vi "FloatingMean_Example.vi"() -> ()   [LabVIEW 2019]
doc: "This example shows how to compute and show a floating mean live image.\nHere the camera class is operated in fifo mode to always get next image in buffer.\nThe Average Count defines the number of images that will be averaged.\nAveraging is done by fetiching one image and using average image from previous iteration\n(avg_n = (1-1/avg_count)*avg_(n-1) + (1/avg_count)*image_n)\n\nIt is a good starting point for writing own applications.\nBut it will not be fail save, i.e. doesnt react on errors, just handles them forward to the end\n\nUsage:\nSelect your required fifo buffer size and image format and start the program.\nOnce started, the camera class will be initialized and image record will start automatically.\nInside the acquisition loop the program calculates the floating average image shows it.\nThe average count can be changed at any time.\nBy using the ROI parameters you can crop the image to select certain regions\n\nBy clicking Quit Application the record will stop and will force an exit of the camera class"
uses:
  camera/Camera.lvclass
  <vilib>/picture/picture.llb/Draw True-Color Pixmap.vi
  <vilib>/picture/picture.llb/Draw 8-Bit Pixmap.vi
panel:
  out "colormap(U8)":u32[](array[numeric])
  in  "Zoom [%]":i32(slide)=26 min=10 max=200 step=5 scale=10.0..200.0
  out "Image":picture
  out "Image(U16)":u16[][](graph)
  in  "averageCount":u8=10 caption="Average Count" min=2
  in  "data_format":T1(ring)=enum."Mono16"
  out "Recorded Images":u32
  in  "Quit":bool
  in  "cropY1":u64=2048 min=1 max=2048 step=1
  in  "cropX1":u64=2048 min=1 max=2048 step=1
  in  "cropY0":u64=1 min=1 max=2047 step=1
  in  "cropX0":u64=1 min=1 max=2047 step=1
  out "Image Height":u64
  out "Image Width":u64
  in  "dwImgCount":u32=10 caption="Fifo Buffer Size" max=4023
  out "Error":errorcluster {"code" format="%x"}
  # "This example shows how to compute and show a floating mean live image.\nHere the camera class is operated in fifo mode to always get next image in buffer.\nThe Average Count defines the number of images that will be averaged.\nAveraging is done by fetiching one image and using average image from previous iteration\n(avg_n = (1-1/avg_count)*avg_(n-1) + (1/avg_count)*image_n)\n\nIt is a good starting point for writing own applications.\nBut it will not be fail save, i.e. doesnt react on errors, just handles them forward to the end\n\nUsage:\nSelect your required fifo buffer size and image format and start the program.\nOnce started, the camera class will be initialized and image record will start automatically.\nInside the acquisition loop the program calculates the floating average image shows it.\nThe average count can be changed at any time.\nBy using the crop parameters you can crop the image to select certain regions\n\nBy clicking Quit Application the record will stop and will force an exit of the camera class"
  # "pco.labview"
  # "Camera Setup"
  # "Recording Control"
  # "Parameters for image readout"
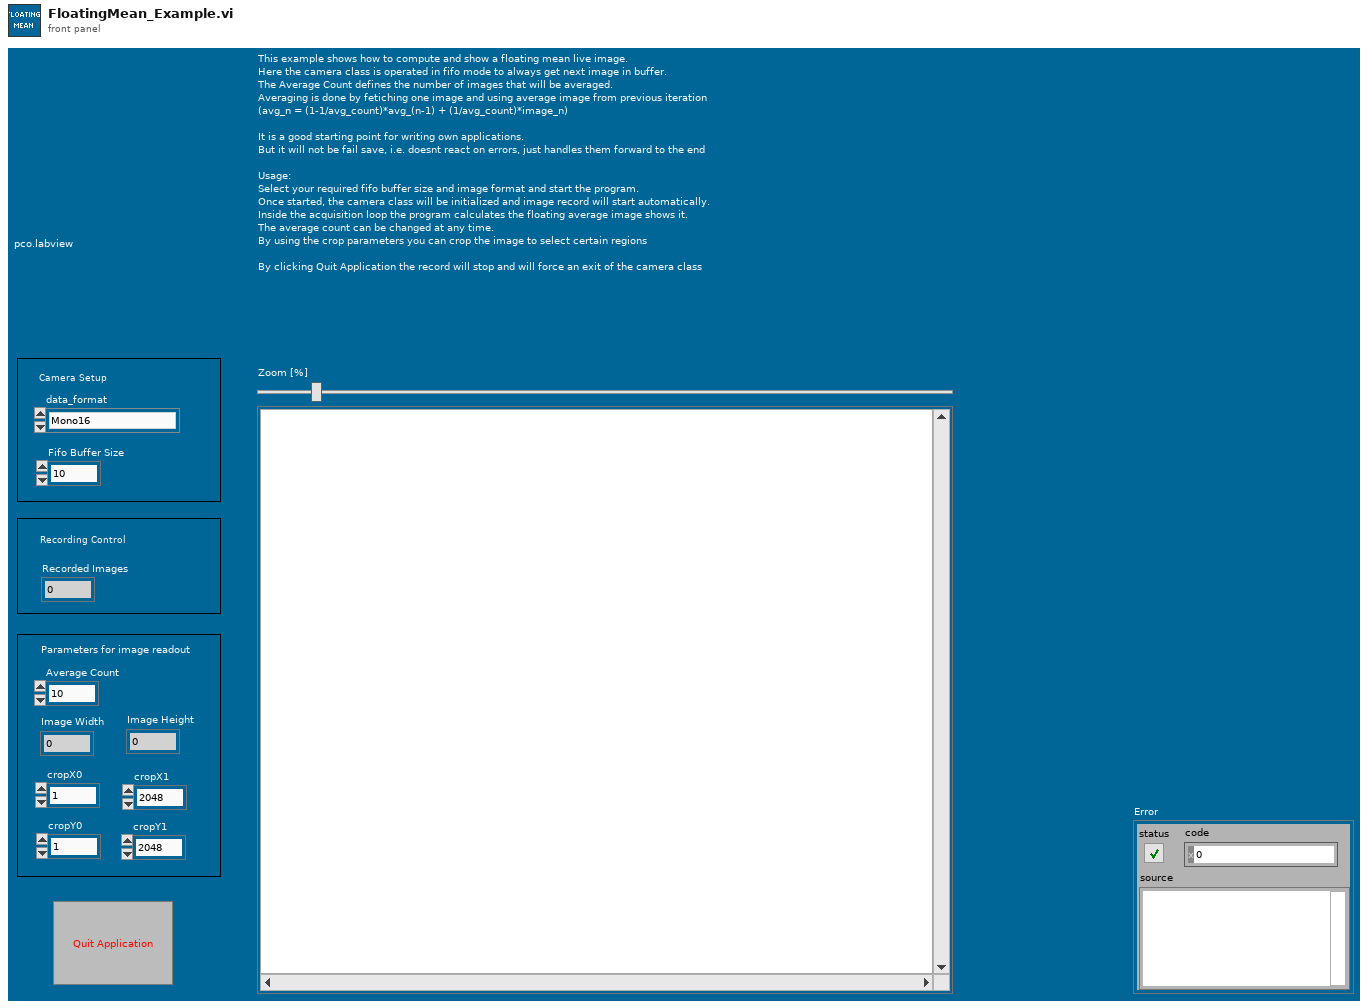
[diagram p1: front panel]
types:
  T1 = enum16{"Undefined", "Mono8", "Mono16", "BGRA8", "RGBA8", "BGRA16", "RGBA16", "CompressedMono8"}
  T2 = enum8{"Enabled", "Disabled", "Disabled and Grayed Out"}
  T3 = enum16{"sequence", "sequence non blocking", "ring buffer", "fifo", "tif", "multitif", "pcoraw", "b16", "dicom", "multidicom", "camram_ring", "camram_segment"}
  T4 = typedef "Camera.lvclass/binning.ctl" = cluster{"vert":u16, "horz":u16, "mode":u16}
  T5 = cluster{"exposure_time_s":dbl, "delay_time_s":dbl, "roi":cluster{"x0":u64, "y0":u64, "x1":u64, "y1":u64}, "timestamp_mode":u16, "pixelrate":u32, "conversion_factor":sgl, "trigger_mode":u16, "acquire_mode":u16, "acquire_sequence_number":u32, "metadata_mode":u16, "noisefilter_mode":u16, "pixel_format":u32, "binning":T4, "auto_exposure":cluster{"region":u16, "min_exposure_s":dbl, "max_exposure_s":dbl}}
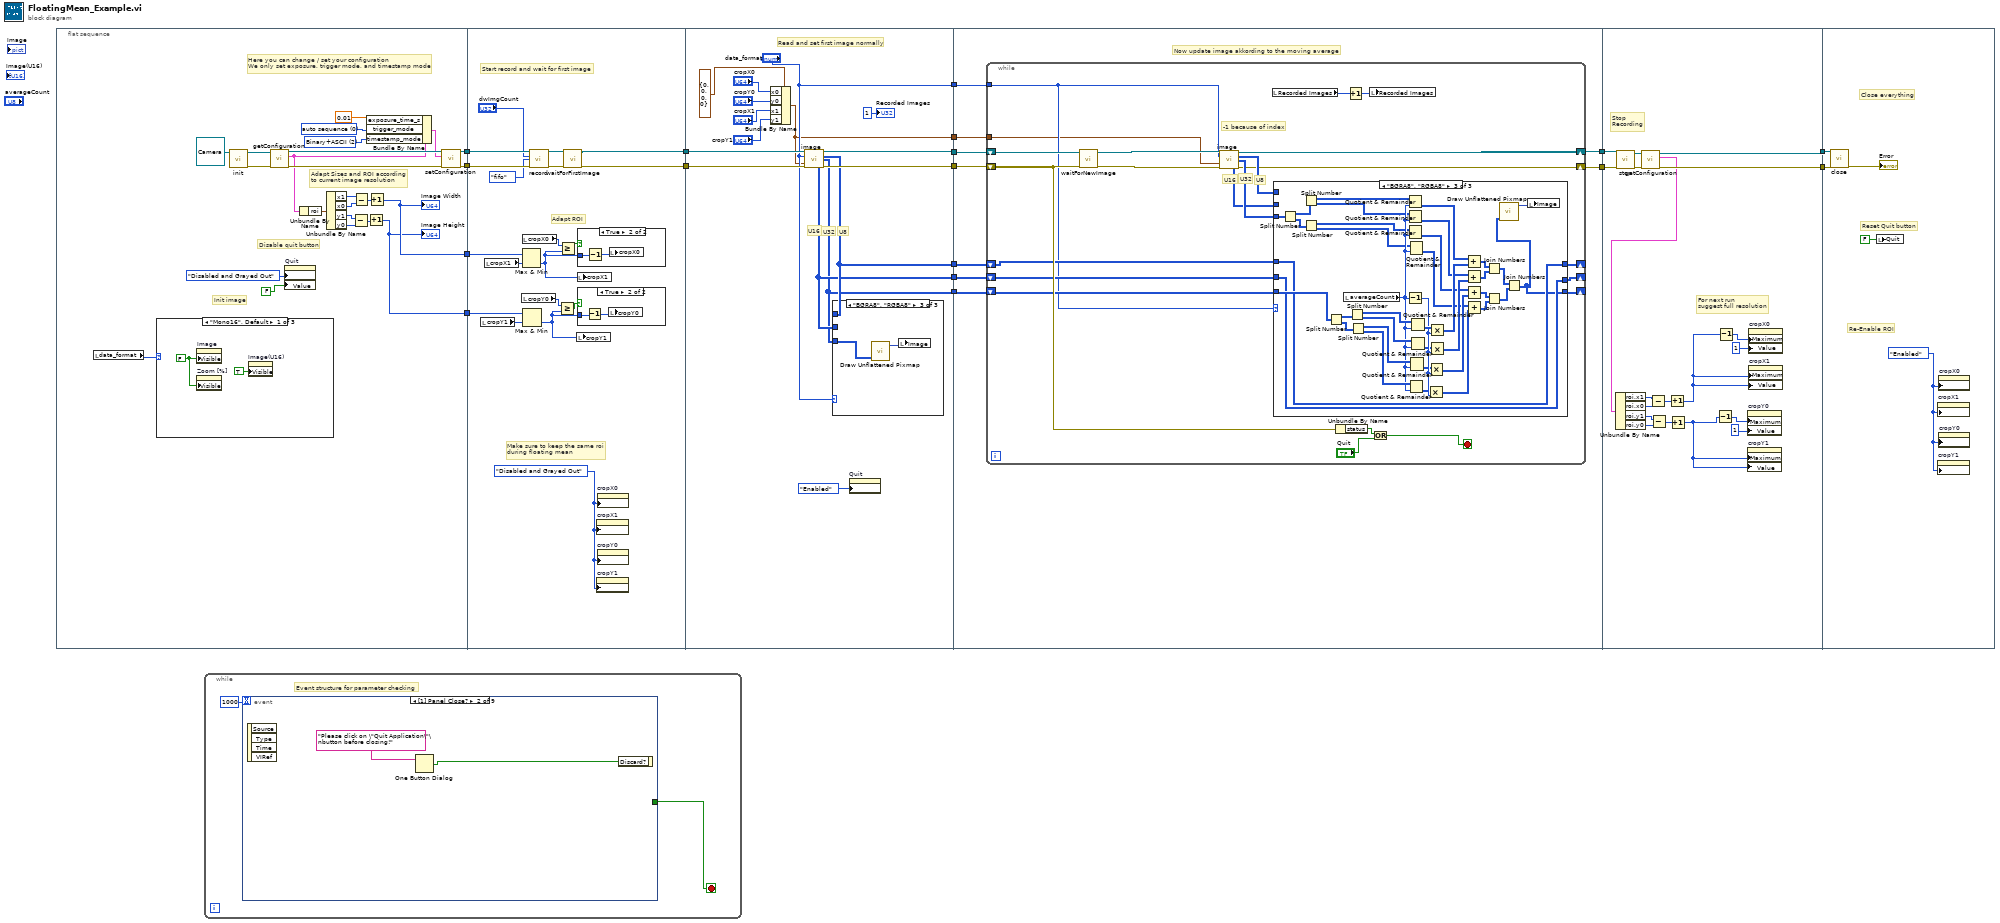
[diagram p0: block diagram]
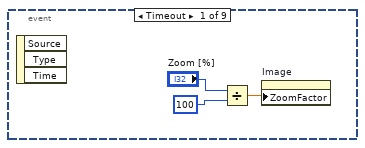
[diagram p2: hidden frame]
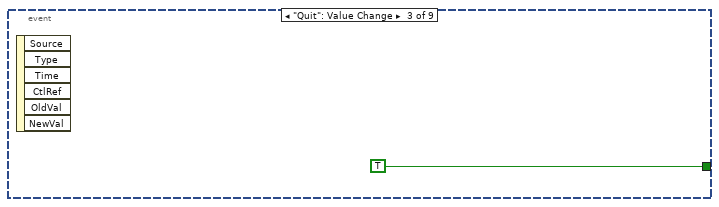
[diagram p3: hidden frame]
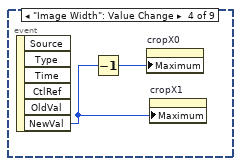
[diagram p4: hidden frame]
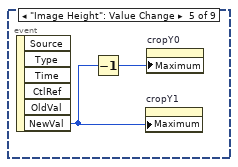
[diagram p5: hidden frame]
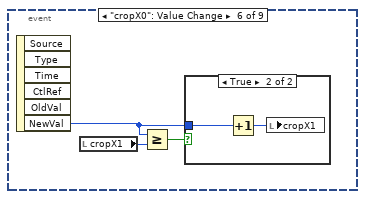
[diagram p6: hidden frame]
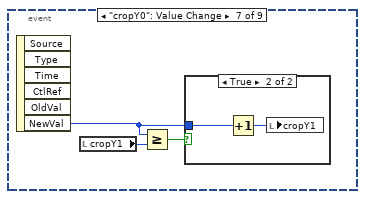
[diagram p8: hidden frame]
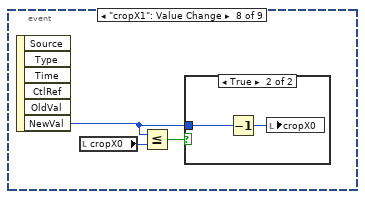
[diagram p10: hidden frame]
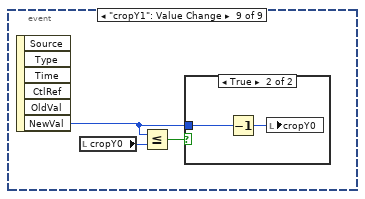
[diagram p12: hidden frame]
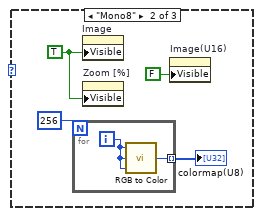
[diagram p14: hidden frame]
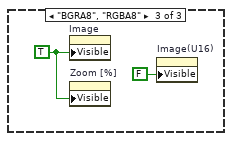
[diagram p15: hidden frame]
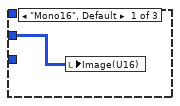
[diagram p18: hidden frame]
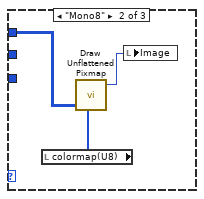
[diagram p19: hidden frame]
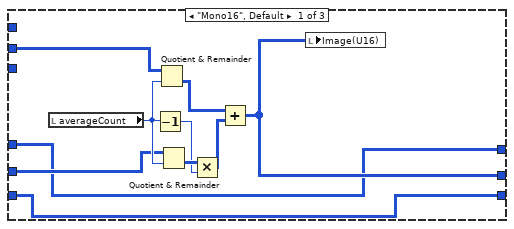
[diagram p20: hidden frame]
diagram:
  n1 = flat-sequence {
    tunnel: [w34] -> w17
    tunnel: [w33] -> w16
    tunnel: [w20] -> w2
    tunnel: [w19] -> w1
    tunnel: w17 -> [w70]
    tunnel: w16 -> [w69]
    tunnel: [w65] -> w15
    tunnel: [w64] -> w14
    tunnel: w2 -> [w54]
    tunnel: w1 -> [w53]
    tunnel: w15 -> [w89]
    tunnel: w14 -> [w88]
    tunnel: [w85] -> w13
    tunnel: [w86] -> w12
    tunnel: ["data_format"] -> w7
    tunnel: [w83] -> w6
    tunnel: [w82] -> w5
    tunnel: [w81] -> w4
    tunnel: [w75] -> w3
    tunnel: w13 -> [w104]
    tunnel: w12 -> [w105]
    tunnel: [w103] -> w11
    tunnel: [w102] -> w9
    tunnel: w7 -> [w101]
    tunnel: w6 -> [w100]
    tunnel: w5 -> [w99]
    tunnel: w4 -> [w98]
    tunnel: w3 -> [w97]
    tunnel: w11 -> [w206]
    tunnel: [w201] -> w10
    tunnel: w9 -> [w205]
    tunnel: [w202] -> w8
    tunnel: w10 -> [w209]
    tunnel: w8 -> [w208]
    frame #0 {
      w24 = u16 2 items=["OFF", "Binary", "Binary+ASCII", "ASCII"] ("TimestampMode")
      w38 = u16 0 items=["auto sequence"=0, "software trigger"=1, "external exposure start & software trigger"=2, "external exposure control"=3, "external synchronized"=4, "fast external exposure control"=5, "external CDS control"=6, "slow external exposure control"=7, "external synchronized HDSDI"=258] ("TriggerMode")
      # "Here you can change / set your configuration\nWe only set exposure, trigger mode, and timestamp mode"
      # "Init image"
      # "Adapt Sizes and ROI according\nto current image resolution"
      # "Disable quit button"
      n2 = local read "data_format"() -> (w21:T1)
      n3 = case shown="\"Mono16\", Default" w21 {
        frame "Mono16", Default {
          w42 = FALSE ("Visible")
          n4 = property on="Image" class="Pict"("Visible"=w42) -> ()  [unwired: 2 in, 2 out]
          n5 = property on="Zoom [%]" class="Slide (strict)"("Visible"=w42) -> ()  [unwired: 2 in, 2 out]
          n6 = property on="Image(U16)" class="IntGraph (strict)"("Visible"=TRUE) -> ()  [unwired: 2 in, 2 out]
        }
        frame "Mono8" {
          w46 = TRUE ("Visible")
          n7 = for {
            N: 256 -> [_]
            tunnel: [w48] -> w45 mode=indexing
            i -> [w49]
            n8 = call <vilib>:"RGB to Color.vi"("B"=w49, "G"=w49, "R"=w49) -> ("Color"=w48:u32)
          }
          "colormap(U8)" <- w45
          n9 = property on="Image" class="Pict"("Visible"=w46) -> ()  [unwired: 2 in, 2 out]
          n10 = property on="Zoom [%]" class="Slide (strict)"("Visible"=w46) -> ()  [unwired: 2 in, 2 out]
          n11 = property on="Image(U16)" class="IntGraph (strict)"("Visible"=FALSE) -> ()  [unwired: 2 in, 2 out]
        }
        frame "BGRA8", "RGBA8" {
          w50 = TRUE ("Visible")
          n12 = property on="Image" class="Pict"("Visible"=w50) -> ()  [unwired: 2 in, 2 out]
          n13 = property on="Zoom [%]" class="Slide (strict)"("Visible"=w50) -> ()  [unwired: 2 in, 2 out]
          n14 = property on="Image(U16)" class="IntGraph (strict)"("Visible"=FALSE) -> ()  [unwired: 2 in, 2 out]
        }
      }
      n15 = call-dynamic "init.vi"("Camera in"=refnum<class "Camera.lvclass"> refnum ("PCOCamera in")) -> ("Camera out"=w40:refnum<class "Camera.lvclass">, "error out"=w39:errorcluster)  [unwired: 8 in]
      n16 = call-dynamic "getConfiguration.vi"("error in (no error)"=w39, "Camera in"=w40) -> ("error out"=w36:errorcluster, "configuration"=w32:T5, "Camera out"=w37:refnum<class "Camera.lvclass">)  [unwired: 7 in]
      n17 = property on="Quit" class="Bool (strict)"("DisabledEnum"=T2."Disabled and Grayed Out" ("Disabled"), "Value"=FALSE ("Stop")) -> ()  [unwired: 2 in, 2 out]
      n18 = Unbundle By Name(w32) -> ("roi"=w31:cluster{"x0":u64, "y0":u64, "x1":u64, "y1":u64})
      n19 = Unbundle By Name(w31) -> ("x1"=w29:u64, "x0"=w30:u64, "y1"=w27:u64, "y0"=w28:u64)
      n20 = Subtract(x=w27, y=w28) -> (x-y=w25:u64)
      n21 = Subtract(x=w29, y=w30) -> (x-y=w26:u64)
      n22 = Bundle By Name(cluster=w32, "exposure_time_s"=0.01, "trigger_mode"=w38, "timestamp_mode"=w24) -> (w35:T5)
      n23 = Increment(x=w25) -> (x+1=w19:u64)
      "Image Height" <- w19
      n24 = Increment(x=w26) -> (x+1=w20:u64)
      "Image Width" <- w20
      n25 = call-dynamic "setConfiguration.vi"("error in (no error)"=w36, "configuration"=w35, "Camera in"=w37) -> ("error out"=w33:errorcluster, "Camera out"=w34:refnum<class "Camera.lvclass">)  [unwired: 7 in]
    }
    frame #1 {
      w63 = T2."Disabled and Grayed Out" ("Disabled")
      # "Adapt ROI"
      # "Make sure to keep the same roi\nduring floating mean"
      # "Start record and wait for first image"
      n26 = local read "cropY1"() -> (w61:u64)
      n27 = local read "cropX1"() -> (w62:u64)
      n28 = local read "cropY0"() -> (w56:u64)
      n29 = local read "cropX0"() -> (w60:u64)
      n30 = Max & Min(x=w54, y=w62) -> (min(x,y)=w58:u64)  [unwired: 1 out]
      n31 = Max & Min(x=w53, y=w61) -> (min(x,y)=w55:u64)  [unwired: 1 out]
      n32 = call-dynamic "record.vi"("Camera in"=w70, "num_images"="dwImgCount", "record_mode"=T3."fifo", "error in (no error)"=w69) -> ("Camera out"=w66:refnum<class "Camera.lvclass">, "error out"=w67:errorcluster)  [unwired: 10 in]
      n33 = Greater Or Equal?(x=w56, y=w55) -> (x >= y?=w57:bool)
      n34 = Greater Or Equal?(x=w60, y=w58) -> (x >= y?=w59:bool)
      n35 = call-dynamic "waitForFirstImage.vi"("error in (no error)"=w67, "Camera in"=w66) -> ("error out"=w64:errorcluster, "Camera out"=w65:refnum<class "Camera.lvclass">)  [unwired: 8 in]
      n36 = local write "cropY1"(w55) -> ()
      n37 = local write "cropX1"(w58) -> ()
      n38 = case shown="True" w57 {
        tunnel: w55 -> [_ w72]
        frame False {
        }
        frame True {
          n39 = Decrement(x=w72) -> (x-1=w71:u64)
          n40 = local write "cropY0"(w71) -> ()
        }
      }
      n41 = case shown="True" w59 {
        tunnel: w58 -> [_ w74]
        frame False {
        }
        frame True {
          n42 = Decrement(x=w74) -> (x-1=w73:u64)
          n43 = local write "cropX0"(w73) -> ()
        }
      }
      n44 = property on="cropX1" class="DigNum (strict)"("DisabledEnum"=w63) -> ()  [unwired: 2 in, 2 out]
      n45 = property on="cropY1" class="DigNum (strict)"("DisabledEnum"=w63) -> ()  [unwired: 2 in, 2 out]
      n46 = property on="cropX0" class="DigNum (strict)"("DisabledEnum"=w63) -> ()  [unwired: 2 in, 2 out]
      n47 = property on="cropY0" class="DigNum (strict)"("DisabledEnum"=w63) -> ()  [unwired: 2 in, 2 out]
    }
    frame #2 {
      # "U32"
      # "U8"
      # "U16"
      # "Read and set first image normally"
      n48 = Bundle By Name(cluster=cluster{"x0":u64, "y0":u64, "x1":u64, "y1":u64} {"x0"=0, "y0"=0, "x1"=0, "y1"=0} ("roi"), "x0"="cropX0", "y0"="cropY0", "x1"="cropX1", "y1"="cropY1") -> (w75:cluster{"x0":u64, "y0":u64, "x1":u64, "y1":u64})
      n49 = call-dynamic "image.vi"("Camera in"=w89, "data_format"="data_format", "crop"=w75, "error in (no error)"=w88) -> ("Camera out"=w85:refnum<class "Camera.lvclass">, "image (U8)"=w83:u8[][], "image (U32)"=w81:u32[][], "raw_image (U16)"=w82:u16[][], "error out"=w86:errorcluster)  [unwired: 3 in, 4 out]
      n50 = case shown="\"BGRA8\", \"RGBA8\"" "data_format" {
        tunnel: w81 -> [_ _ w96]
        tunnel: w83 -> [_ w94 _]
        tunnel: w82 -> [w91 _ _]
        frame "Mono16", Default {
          n51 = local write "Image(U16)"(w91) -> ()
        }
        frame "Mono8" {
          n52 = local read "colormap(U8)"() -> (w92:u32[])
          n53 = call-poly <vilib>:"Draw Unflattened Pixmap.vi"("data"=w94, "color table"=w92) -> ("new picture"=w93:picture)  [unwired: 7 in]
          n54 = local write "Image"(w93) -> ()
        }
        frame "BGRA8", "RGBA8" {
          n55 = call-poly <vilib>:"Draw Unflattened Pixmap.vi"("data (RGB format)"=w96) -> ("new picture"=w95:picture)  [unwired: 8 in]
          n56 = local write "Image"(w95) -> ()
        }
      }
      n57 = property on="Quit" class="Bool (strict)"("DisabledEnum"=T2."Enabled" ("Disabled")) -> ()  [unwired: 2 in, 2 out]
      "Recorded Images" <- u32 1 ("Recorded Images")
    }
    frame #3 {
      # "Now update image akkording to the moving average"
      n58 = while {
        shift-right: [w127] -> w103
        shift-left: w104 -> [w126]
        shift-right: [w107] -> w102
        shift-left: w105 -> [w121]
        tunnel: w101 -> [w110]
        shift-right: [w113] -> _
        shift-left: w100 -> [w117]
        shift-right: [w111] -> _
        shift-left: w99 -> [w116]
        shift-right: [w112] -> _
        shift-left: w98 -> [w115]
        tunnel: w97 -> [w106]
        stop <- w118 stop-if-true
        # "U8"
        # "-1 because of index"
        # "U32"
        # "U16"
        n59 = call-dynamic "waitForNewImage.vi"("error in (no error)"=w121, "Camera in"=w126) -> ("error out"=w122:errorcluster, "Camera out"=w123:refnum<class "Camera.lvclass">)  [unwired: 8 in]
        n60 = call-dynamic "image.vi"("Camera in"=w123, "data_format"=w110, "crop"=w106, "error in (no error)"=w122) -> ("Camera out"=w127:refnum<class "Camera.lvclass">, "image (U8)"=w114:u8[][], "image (U32)"=w109:u32[][], "raw_image (U16)"=w108:u16[][], "error out"=w107:errorcluster)  [unwired: 3 in, 4 out]
        n61 = local read "Recorded Images"() -> (w125:u32)
        n62 = case shown="\"BGRA8\", \"RGBA8\"" w110 {
          tunnel: w109 -> [_ _ w153]
          tunnel: w108 -> [w133 _ _]
          tunnel: w117 -> [w130 w147 w151]
          tunnel: w116 -> [w132 w139 w152]
          tunnel: w115 -> [w129 w138 w186]
          tunnel: w114 -> [_ w143 _]
          tunnel: [w130 w140 w151] -> w113
          tunnel: [w129 w138 w150] -> w112
          tunnel: [w131 w139 w152] -> w111
          frame "Mono16", Default {
            n63 = local read "averageCount"() -> (w136:u8)
            n64 = Decrement(x=w136) -> (x-1=w128:u8)
            n65 = Quotient & Remainder(x=w133, y=w136) -> (floor(x/y)=w135:u16[][])  [unwired: 1 out]
            n66 = Quotient & Remainder(x=w132, y=w136) -> (floor(x/y)=w137:u16[][])  [unwired: 1 out]
            n67 = Multiply(x=w137, y=w128) -> (x*y=w134:u16[][])
            n68 = Add(x=w135, y=w134) -> (x+y=w131:u16[][])
            n69 = local write "Image(U16)"(w131) -> ()
          }
          frame "Mono8" {
            n70 = local read "averageCount"() -> (w144:u8)
            n71 = Decrement(x=w144) -> (x-1=w145:u8)
            n72 = Quotient & Remainder(x=w143, y=w144) -> (floor(x/y)=w142:u8[][])  [unwired: 1 out]
            n73 = Quotient & Remainder(x=w147, y=w144) -> (floor(x/y)=w146:u8[][])  [unwired: 1 out]
            n74 = Multiply(x=w146, y=w145) -> (x*y=w141:u8[][])
            n75 = Add(x=w142, y=w141) -> (x+y=w140:u8[][])
            n76 = local read "colormap(U8)"() -> (w148:u32[])
            n77 = call-poly <vilib>:"Draw Unflattened Pixmap.vi"("data"=w140, "color table"=w148) -> ("new picture"=w149:picture)  [unwired: 7 in]
            n78 = local write "Image"(w149) -> ()
          }
          frame "BGRA8", "RGBA8" {
            n79 = Split Number(x=w153) -> (hi(x)=w174:u16[][], lo(x)=w173:u16[][])
            n80 = Split Number(x=w174) -> (hi(x)=w171:u8[][], lo(x)=w170:u8[][])
            n81 = Split Number(x=w173) -> (hi(x)=w169:u8[][], lo(x)=w168:u8[][])
            n82 = Split Number(x=w186) -> (hi(x)=w185:u16[][], lo(x)=w184:u16[][])
            n83 = local read "averageCount"() -> (w172:u8)
            n84 = Split Number(x=w185) -> (hi(x)=w182:u8[][], lo(x)=w177:u8[][])
            n85 = Split Number(x=w184) -> (hi(x)=w176:u8[][], lo(x)=w175:u8[][])
            n86 = Quotient & Remainder(x=w171, y=w172) -> (floor(x/y)=w167:u8[][])  [unwired: 1 out]
            n87 = Quotient & Remainder(x=w170, y=w172) -> (floor(x/y)=w165:u8[][])  [unwired: 1 out]
            n88 = Quotient & Remainder(x=w169, y=w172) -> (floor(x/y)=w161:u8[][])  [unwired: 1 out]
            n89 = Decrement(x=w172) -> (x-1=w181:u8)
            n90 = Quotient & Remainder(x=w168, y=w172) -> (floor(x/y)=w160:u8[][])  [unwired: 1 out]
            n91 = Quotient & Remainder(x=w175, y=w172) -> (floor(x/y)=w180:u8[][])  [unwired: 1 out]
            n92 = Quotient & Remainder(x=w176, y=w172) -> (floor(x/y)=w179:u8[][])  [unwired: 1 out]
            n93 = Quotient & Remainder(x=w182, y=w172) -> (floor(x/y)=w183:u8[][])  [unwired: 1 out]
            n94 = Quotient & Remainder(x=w177, y=w172) -> (floor(x/y)=w178:u8[][])  [unwired: 1 out]
            n95 = Multiply(x=w180, y=w181) -> (x*y=w162:u8[][])
            n96 = Multiply(x=w179, y=w181) -> (x*y=w163:u8[][])
            n97 = Multiply(x=w183, y=w181) -> (x*y=w166:u8[][])
            n98 = Multiply(x=w178, y=w181) -> (x*y=w164:u8[][])
            n99 = Add(x=w167, y=w166) -> (x+y=w159:u8[][])
            n100 = Add(x=w165, y=w164) -> (x+y=w158:u8[][])
            n101 = Add(x=w161, y=w163) -> (x+y=w157:u8[][])
            n102 = Add(x=w160, y=w162) -> (x+y=w156:u8[][])
            n103 = Join Numbers(hi=w159, lo=w158) -> ((hi.lo)=w155:u16[][])
            n104 = Join Numbers(hi=w157, lo=w156) -> ((hi.lo)=w154:u16[][])
            n105 = Join Numbers(hi=w155, lo=w154) -> ((hi.lo)=w150:u32[][])
            n106 = call-poly <vilib>:"Draw Unflattened Pixmap.vi"("data (RGB format)"=w150) -> ("new picture"=w187:picture)  [unwired: 8 in]
            n107 = local write "Image"(w187) -> ()
          }
        }
        n108 = Unbundle By Name(w121) -> ("status"=w120:bool)
        n109 = Increment(x=w125) -> (x+1=w124:u32)
        n110 = local write "Recorded Images"(w124) -> ()
        n111 = Or(x=w120, y="Quit") -> (x .or. y?=w118:bool)
      }
    }
    frame #4 {
      # "For next run \nsuggest full resolution"
      # "Stop \nRecording"
      n112 = call-dynamic "stop.vi"("error in (no error)"=w205, "Camera in"=w206) -> ("error out"=w203:errorcluster, "Camera out"=w204:refnum<class "Camera.lvclass">)  [unwired: 8 in]
      n113 = call-dynamic "getConfiguration.vi"("error in (no error)"=w203, "Camera in"=w204) -> ("error out"=w202:errorcluster, "configuration"=w200:T5, "Camera out"=w201:refnum<class "Camera.lvclass">)  [unwired: 7 in]
      n114 = Unbundle By Name(w200) -> ("roi.x1"=w194:u64, "roi.x0"=w195:u64, "roi.y1"=w196:u64, "roi.y0"=w197:u64)
      n115 = Subtract(x=w194, y=w195) -> (x-y=w193:u64)
      n116 = Subtract(x=w196, y=w197) -> (x-y=w192:u64)
      n117 = Increment(x=w193) -> (x+1=w189:u64)
      n118 = Increment(x=w192) -> (x+1=w190:u64)
      n119 = Decrement(x=w190) -> (x-1=w191:u64)
      n120 = Decrement(x=w189) -> (x-1=w188:u64)
      n121 = property on="cropY0" class="DigNum (strict)"("Maximum"=w191, "Value"=u64 1 ("roiY0")) -> ()  [unwired: 2 in, 2 out]
      n122 = property on="cropY1" class="DigNum (strict)"("Maximum"=w190, "Value"=w190) -> ()  [unwired: 2 in, 2 out]
      n123 = property on="cropX0" class="DigNum (strict)"("Maximum"=w188, "Value"=u64 1 ("roiX0")) -> ()  [unwired: 2 in, 2 out]
      n124 = property on="cropX1" class="DigNum (strict)"("Maximum"=w189, "Value"=w189) -> ()  [unwired: 2 in, 2 out]
    }
    frame #5 {
      w207 = T2."Enabled" ("Disabled")
      # "Re-Enable ROI"
      # "Reset Quit button"
      # "Close everything"
      n125 = call-dynamic "close.vi"("error in (no error)"=w208, "Camera in"=w209) -> ("error out"=→"Error":errorcluster)  [unwired: 9 in]
      n126 = local write "Quit"(FALSE ("Stop")) -> ()
      n127 = property on="cropX1" class="DigNum (strict)"("DisabledEnum"=w207) -> ()  [unwired: 2 in, 2 out]
      n128 = property on="cropY1" class="DigNum (strict)"("DisabledEnum"=w207) -> ()  [unwired: 2 in, 2 out]
      n129 = property on="cropX0" class="DigNum (strict)"("DisabledEnum"=w207) -> ()  [unwired: 2 in, 2 out]
      n130 = property on="cropY0" class="DigNum (strict)"("DisabledEnum"=w207) -> ()  [unwired: 2 in, 2 out]
    }
  }
  n131 = while {
    stop <- w212 stop-if-true
    # "Event structure for parameter checking"
    n132 = event shown="[1] Panel Close?" {
      selector: _ -> [_ _ _ _ _ _ _ _ _]
      dyn-events: _ -> [_ _ _ _ _ _ _ _ _]
      timeout: 1000 -> [_ _ _ _ _ _ _ _ _]
      tunnel: [_ _ TRUE _ _ _ _ _ _] -> w212
      event Timeout {
        n133 = event-data() -> ()  [unwired: 1 in, 3 out]
        n134 = Divide(x="Zoom [%]", y=100 ("Zoom [%]")) -> (x/y=w216:dbl)
        n135 = property on="Image" class="Pict"("ZoomFactor"=w216) -> ()  [unwired: 2 in, 2 out]
      }
      event Panel Close? {
        n136 = event-data() -> ()  [unwired: 1 in, 4 out]
        n137 = One Button Dialog(message="Please click on \"Quit Application\"\nbutton before closing!") -> (true=w217:bool)  [unwired: 1 in]
        n138 = event-data("Discard?"=w217) -> ()  [unwired: 1 in, 1 out]
      }
      event "Quit": Value Change {
        n139 = event-data() -> ()  [unwired: 1 in, 6 out]
      }
      event "Image Width": Value Change {
        n140 = event-data() -> ("NewVal"=w220:u64)  [unwired: 1 in, 5 out]
        n141 = Decrement(x=w220) -> (x-1=w221:u64)
        n142 = property on="cropX0" class="DigNum (strict)"("Maximum"=w221) -> ()  [unwired: 2 in, 2 out]
        n143 = property on="cropX1" class="DigNum (strict)"("Maximum"=w220) -> ()  [unwired: 2 in, 2 out]
      }
      event "Image Height": Value Change {
        n144 = event-data() -> ("NewVal"=w222:u64)  [unwired: 1 in, 5 out]
        n145 = Decrement(x=w222) -> (x-1=w223:u64)
        n146 = property on="cropY1" class="DigNum (strict)"("Maximum"=w222) -> ()  [unwired: 2 in, 2 out]
        n147 = property on="cropY0" class="DigNum (strict)"("Maximum"=w223) -> ()  [unwired: 2 in, 2 out]
      }
      event "cropX0": Value Change {
        n148 = event-data() -> ("NewVal"=w224:u64)  [unwired: 1 in, 5 out]
        n149 = local read "cropX1"() -> (w226:u64)
        n150 = Greater Or Equal?(x=w224, y=w226) -> (x >= y?=w225:bool)
        n151 = case shown="True" w225 {
          tunnel: w224 -> [_ w228]
          frame False {
          }
          frame True {
            n152 = Increment(x=w228) -> (x+1=w227:u64)
            n153 = local write "cropX1"(w227) -> ()
          }
        }
      }
      event "cropY0": Value Change {
        n154 = event-data() -> ("NewVal"=w229:u64)  [unwired: 1 in, 5 out]
        n155 = local read "cropY1"() -> (w231:u64)
        n156 = Greater Or Equal?(x=w229, y=w231) -> (x >= y?=w230:bool)
        n157 = case shown="True" w230 {
          tunnel: w229 -> [_ w233]
          frame False {
          }
          frame True {
            n158 = Increment(x=w233) -> (x+1=w232:u64)
            n159 = local write "cropY1"(w232) -> ()
          }
        }
      }
      event "cropX1": Value Change {
        n160 = event-data() -> ("NewVal"=w234:u64)  [unwired: 1 in, 5 out]
        n161 = local read "cropX0"() -> (w236:u64)
        n162 = Less Or Equal?(x=w234, y=w236) -> (x <= y?=w235:bool)
        n163 = case shown="True" w235 {
          tunnel: w234 -> [_ w238]
          frame False {
          }
          frame True {
            n164 = Decrement(x=w238) -> (x-1=w237:u64)
            n165 = local write "cropX0"(w237) -> ()
          }
        }
      }
      event "cropY1": Value Change {
        n166 = event-data() -> ("NewVal"=w239:u64)  [unwired: 1 in, 5 out]
        n167 = local read "cropY0"() -> (w241:u64)
        n168 = Less Or Equal?(x=w239, y=w241) -> (x <= y?=w240:bool)
        n169 = case shown="True" w240 {
          tunnel: w239 -> [_ w243]
          frame False {
          }
          frame True {
            n170 = Decrement(x=w243) -> (x-1=w242:u64)
            n171 = local write "cropY0"(w242) -> ()
          }
        }
      }
    }
  }
